vi "Sort Points.vi"(11 "Triangle":T5={"Vertex 1"={"Position"={"x"=0.0, "y"=0.0, "z"=0.0}, "UV"={"u"=0.0, "v"=0.0}, "Colour"=12517256}, "Vertex 2"={"Position"={"x"=0.0, "y"=0.0, "z"=0.0}, "UV"={"u"=0.0, "v"=0.0}, "Colour"=12517256}, "Vertex 3"={"Position"={"x"=0.0, "y"=0.0, "z"=0.0}, "UV"={"u"=0.0, "v"=0.0}, "Colour"=12517256}, "Colour"=0} {"Vertex 3"."UV"."v" min=0 max=1 step=0.1; "Vertex 3"."UV"."u" min=0 max=1 step=0.1; "Vertex 2"."UV"."v" min=0 max=1 step=0.1; "Vertex 2"."UV"."u" min=0 max=1 step=0.1; "Vertex 1"."UV"."v" min=0 max=1 step=0.1; "Vertex 1"."UV"."u" min=0 max=1 step=0.1}) -> (3 "Sorted Triangle":T1={"Top Vertex"={"Position"={"x"=0.0, "y"=0.0, "z"=0.0}, "UV"={"u"=0.0, "v"=0.0}, "Colour"=12517256}, "Mid Vertex"={"Position"={"x"=0.0, "y"=0.0, "z"=0.0}, "UV"={"u"=0.0, "v"=0.0}, "Colour"=12517256}, "Bottom Vertex"={"Position"={"x"=0.0, "y"=0.0, "z"=0.0}, "UV"={"u"=0.0, "v"=0.0}, "Colour"=12517256}, "Colour"=0} {"Bottom Vertex"."UV"."v" min=0 max=1 step=0.1; "Bottom Vertex"."UV"."u" min=0 max=1 step=0.1; "Mid Vertex"."UV"."v" min=0 max=1 step=0.1; "Mid Vertex"."UV"."u" min=0 max=1 step=0.1; "Top Vertex"."UV"."v" min=0 max=1 step=0.1; "Top Vertex"."UV"."u" min=0 max=1 step=0.1})   [LabVIEW 2020, in "Raster (FPGA).lvlib"]
uses:
  Raster (FPGA).lvlib
  Triangle.ctl
  Vertex.ctl
  Vector 3D.ctl
  UV.ctl
  Triangle (Sorted).ctl
  Round SGL.vi
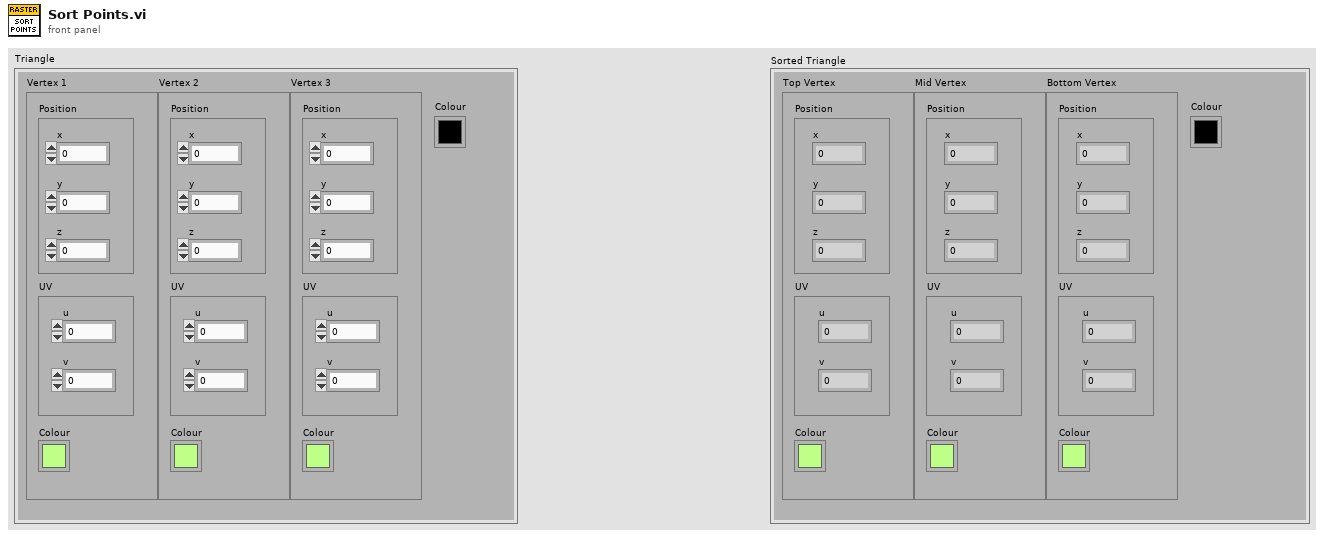
[diagram p1: front panel]
types:
  T1 = typedef "Raster (FPGA).lvlib/Triangle (Sorted).ctl" = cluster{"Top Vertex":T2, "Mid Vertex":T2, "Bottom Vertex":T2, "Colour":u32}
  T2 = typedef "Raster (FPGA).lvlib/Vertex.ctl" = cluster{"Position":T3, "UV":T4, "Colour":u32}
  T3 = typedef "Raster (FPGA).lvlib/Vector 3D.ctl" = cluster{"x":sgl, "y":sgl, "z":sgl}
  T4 = typedef "Raster (FPGA).lvlib/UV.ctl" = cluster{"u":sgl, "v":sgl}
  T5 = typedef "Raster (FPGA).lvlib/Triangle.ctl" = cluster{"Vertex 1":T2, "Vertex 2":T2, "Vertex 3":T2, "Colour":u32}
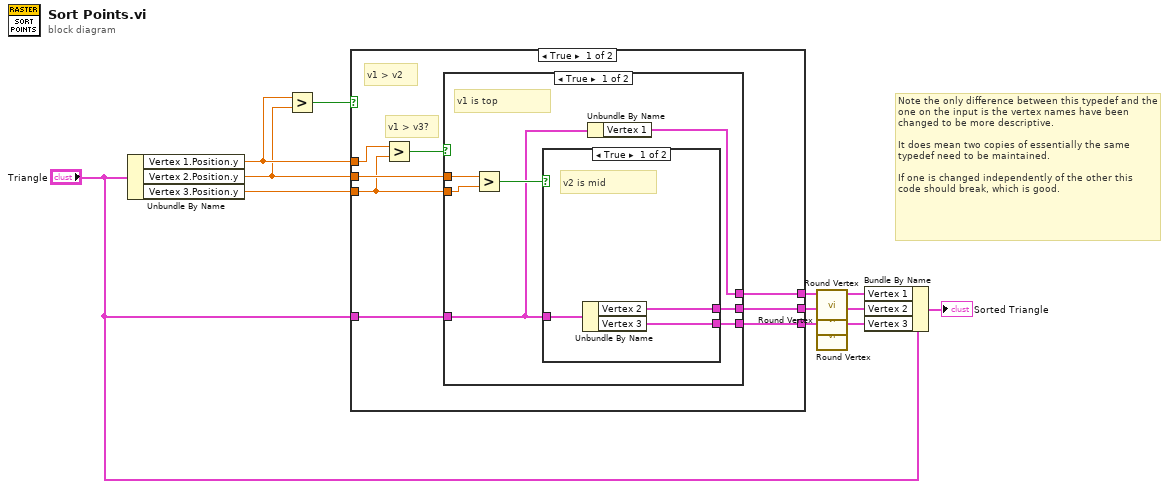
[diagram p0: block diagram]
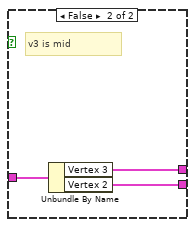
[diagram p2: hidden frame]
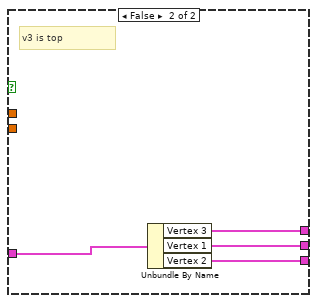
[diagram p3: hidden frame]
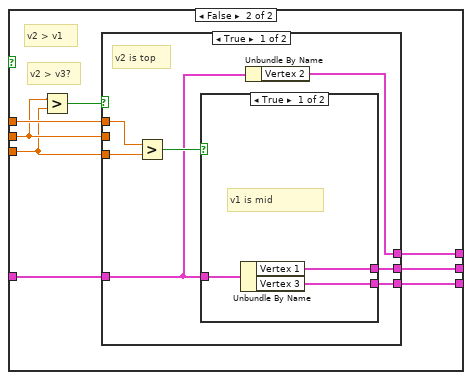
[diagram p4: hidden frame]
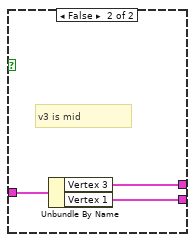
[diagram p5: hidden frame]
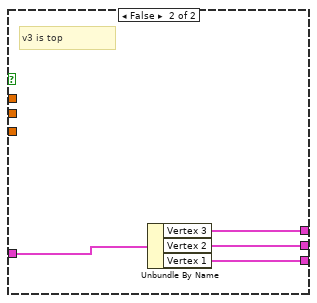
[diagram p6: hidden frame]
diagram:
  # "Note the only difference between this typedef and the one on the input is the vertex names have been changed to be more descriptive.\n\nIt does mean two copies of essentially the same typedef need to be maintained.\n\nIf one is changed independently of the other this code should break, which is good."
  n1 = Unbundle By Name("Triangle") -> ("Vertex 1.Position.y"=w11:sgl, "Vertex 2.Position.y"=w10:sgl, "Vertex 3.Position.y"=w9:sgl)
  n2 = Greater?(x=w11, y=w10) -> (0:w12:bool)
  n3 = case shown="True" w12 {
    tunnel: w11 -> [w20 w40]
    tunnel: w10 -> [w18 w39]
    tunnel: w9 -> [w13 w38]
    tunnel: "Triangle" -> [w17 w44]
    tunnel: [w16 w43] -> w8
    tunnel: [w15 w42] -> w7
    tunnel: [w14 w41] -> w6
    frame True {
      # "v1 > v3?"
      # "v1 > v2"
      n4 = Greater?(x=w20, y=w13) -> (0:w19:bool)
      n5 = case shown="True" w19 {
        tunnel: w18 -> [w27 _]
        tunnel: w13 -> [w26 _]
        tunnel: w17 -> [w22 w35]
        tunnel: [w21 w34] -> w16
        tunnel: [w24 w37] -> w15
        tunnel: [w23 w36] -> w14
        frame True {
          # "v1 is top"
          n6 = Greater?(x=w27, y=w26) -> (0:w25:bool)
          n7 = case shown="True" w25 {
            tunnel: w22 -> [w30 w33]
            tunnel: [w29 w32] -> w24
            tunnel: [w28 w31] -> w23
            frame True {
              # "v2 is mid"
              n8 = Unbundle By Name(w30) -> ("Vertex 2"=w29:T2, "Vertex 3"=w28:T2)
            }
            frame False {
              # "v3 is mid"
              n9 = Unbundle By Name(w33) -> ("Vertex 3"=w32:T2, "Vertex 2"=w31:T2)
            }
          }
          n10 = Unbundle By Name(w22) -> ("Vertex 1"=w21:T2)
        }
        frame False {
          # "v3 is top"
          n11 = Unbundle By Name(w35) -> ("Vertex 3"=w34:T2, "Vertex 1"=w37:T2, "Vertex 2"=w36:T2)
        }
      }
    }
    frame False {
      # "v2 > v3?"
      # "v2 > v1"
      n12 = Greater?(x=w39, y=w38) -> (0:w45:bool)
      n13 = case shown="True" w45 {
        tunnel: w39 -> [_ _]
        tunnel: w38 -> [w52 _]
        tunnel: w44 -> [w48 w60]
        tunnel: [w47 w59] -> w43
        tunnel: [w50 w62] -> w42
        tunnel: [w49 w61] -> w41
        tunnel: w40 -> [w46 _]
        frame True {
          # "v2 is top"
          n14 = Greater?(x=w46, y=w52) -> (0:w51:bool)
          n15 = case shown="True" w51 {
            tunnel: w48 -> [w55 w58]
            tunnel: [w54 w57] -> w50
            tunnel: [w53 w56] -> w49
            frame True {
              # "v1 is mid"
              n16 = Unbundle By Name(w55) -> ("Vertex 1"=w54:T2, "Vertex 3"=w53:T2)
            }
            frame False {
              # "v3 is mid"
              n17 = Unbundle By Name(w58) -> ("Vertex 3"=w57:T2, "Vertex 1"=w56:T2)
            }
          }
          n18 = Unbundle By Name(w48) -> ("Vertex 2"=w47:T2)
        }
        frame False {
          # "v3 is top"
          n19 = Unbundle By Name(w60) -> ("Vertex 3"=w59:T2, "Vertex 2"=w62:T2, "Vertex 1"=w61:T2)
        }
      }
    }
  }
  n20 = call "Round Vertex.vi"("Vertex in"=w8) -> ("Vertex With Position Rounded"=w3:T2)  [unwired: 10 in]
  n21 = call "Round Vertex.vi"("Vertex in"=w7) -> ("Vertex With Position Rounded"=w2:T2)  [unwired: 10 in]
  n22 = call "Round Vertex.vi"("Vertex in"=w6) -> ("Vertex With Position Rounded"=w1:T2)  [unwired: 10 in]
  n23 = Bundle By Name(cluster="Triangle", "Vertex 1"=w3, "Vertex 2"=w2, "Vertex 3"=w1) -> (→"Sorted Triangle":T5)
